vi "Ex6_Secondaire.vi"() -> ()   [LabVIEW 2019]
panel:
  in  "Numeric 2":i16
  in  "Numeric":i32
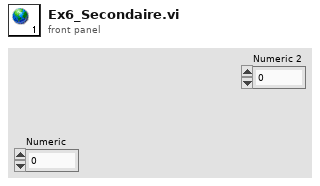
[diagram p1: front panel]
diagram:
